vi "MissingInProjectCLI.vi"   [LabVIEW 2020, in "Missing in Project Tests.lvlib"]
doc: "Provides a command line interface to the Missing In Project test through G-CLI."
uses:
  Missing in Project Tests.lvlib
  <vilib>/Wiresmith Technology/G CLI/CLI Class/CLI.lvclass
  d030f465-a991-474e-afc8-0695029b4070.vi
types:
  T1 = enum16{"open", "replace", "create", "open or create", "replace or create", "replace or create with confirmation"}
  T2 = enum32{"Invalid", "Standard", "Closed", "Hidden", "Minimized", "Maximized"}
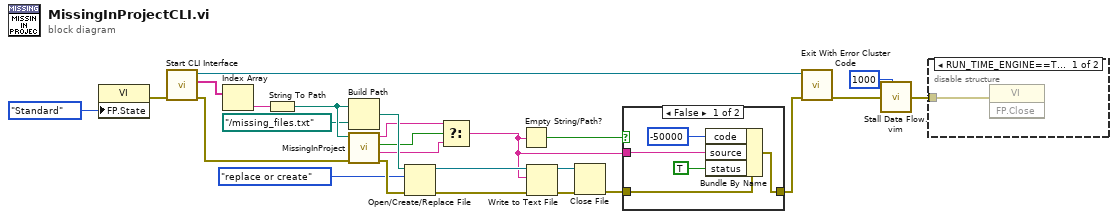
[diagram p0: block diagram]
diagram:
  n1 = property class="VI"("FP.State"=T2."Standard" ("Front Panel Window:State")) -> (error out=w25:errorcluster)  [unwired: 2 in, 1 out]
  n2 = call <vilib>:"Start CLI Interface.vi"("error in (no error)"=w25) -> ("error out"=w24:errorcluster, "Custom Parameters"=w14:string[], "CLI out"=w15:refnum<class "CLI.lvclass">)  [unwired: 7 in, 1 out]
  n3 = Index Array(array=w14) -> (element=w13:string)  [unwired: 1 in]
  n4 = String To Path(string=w13) -> (path=w11:path)
  n5 = Build Path(base path=w11, name or relative path=path "../missing_files.txt") -> (appended path=w9:path)
  n6 = call "MissingInProject.vi"("error in"=w24, "File Path"=w11) -> ("error out"=w21:errorcluster, "Missing Files"=w2:string, "Passed"=w4:bool, "Debug"=w3:string)  [unwired: 6 in]
  n7 = Open/Create/Replace File(file path (use dialog)=w9, error in=w21, operation (0:open)=T1."replace or create") -> (refnum out=w5:refnum<file>, error out=w23:errorcluster)  [unwired: 3 in, 1 out]
  n8 = Select(t=w3, s=w4, f=w2) -> (s? t:f=w1:string)
  n9 = Empty String/Path?(string/path=w1) -> (empty?=w7:bool)
  n10 = Write to Text File(file (use dialog)=w5, text=w1, error in=w23) -> (refnum out=w12:refnum<file>, error out=w22:errorcluster)  [unwired: 1 in, 1 out]
  n11 = Close File(refnum=w12, error in=w22) -> (error out=w20:errorcluster)  [unwired: 1 out]
  n12 = case shown="False" w7 {
    tunnel: w20 -> [w30 w31]
    tunnel: w1 -> [w27 _]
    tunnel: [w29 w31] -> w19
    frame False {
      n13 = Bundle By Name(cluster=w30, "code"=-50000, "source"=w27, "status"=TRUE) -> (w29:errorcluster)
    }
    frame True {
    }
  }
  n14 = call <vilib>:"Exit With Error Cluster Code.vi"("error in (no error)"=w19, "CLI in"=w15) -> ("error out"=w18:errorcluster)  [unwired: 9 in]
  n15 = call "Stall Data Flow.vim"("value in"=w18, "milliseconds to wait"=u32 1000) -> ("value out"=w17:errorcluster)  [unwired: 1 out]
  n16 = disable-structure shown="RUN_TIME_ENGINE==True" {
    disable-tunnel: w17 -> [w32 _]
    frame condition #0 {
      n17 = invoke class="VI" method="FP.Close"(error in=w32) -> ()  [unwired: 2 in, 3 out]
    }
    frame condition #1 (active) {
    }
  }
